vi "Get Default Instrument Configuration.vi"(0 "Instrument Handle In":refnum<k21>) -> (4 "Instrument Handle Out":refnum<k21>, 8 "Instrument Configuration":T1={"LO Sharing Mode"=enum."Automatic", "LO Routing Configurations"=[], "LO Offset Configuration"={"Mode"=enum."Automatic", "Offset (Hz)"=0.0}} {"LO Offset Configuration"."Offset (Hz)" format="%#_6p"})   [LabVIEW 2016, in "RFmxInstr.lvlib"]
uses:
  RFmxInstr.lvlib
  Instrument Configuration.ctl
  Common/Local Oscillator Sharing Mode.ctl
  Common/Local Oscillator Routing Configuration.ctl
  Common/Local Oscillator Frequency Offset Configuration.ctl
  Common/Local Oscillator Frequency Offset Mode.ctl
  <resource>/objmgr/RFmxInstr.rc
  Common/Common.lvlib
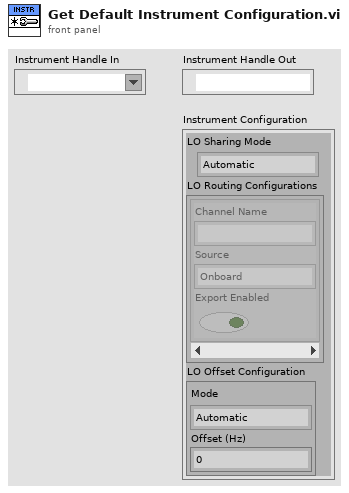
[diagram p1: front panel]
types:
  T1 = typedef "RFmxInstr.lvlib/Instrument Configuration.ctl" = cluster{"LO Sharing Mode":T2, "LO Routing Configurations":T3[], "LO Offset Configuration":T4}
  T2 = typedef "Common.lvlib/Local Oscillator Sharing Mode.ctl" = enum16{"None", "Automatic", "Manual"}
  T3 = typedef "Common.lvlib/Local Oscillator Routing Configuration.ctl" = cluster{"Channel Name":string, "Source":string, "Export Enabled":bool}
  T4 = typedef "Common.lvlib/Local Oscillator Frequency Offset Configuration.ctl" = cluster{"Mode":T5, "Offset (Hz)":dbl}
  T5 = typedef "Common.lvlib/Local Oscillator Frequency Offset Mode.ctl" = enum16{"No Offset", "Automatic", "User Defined"}
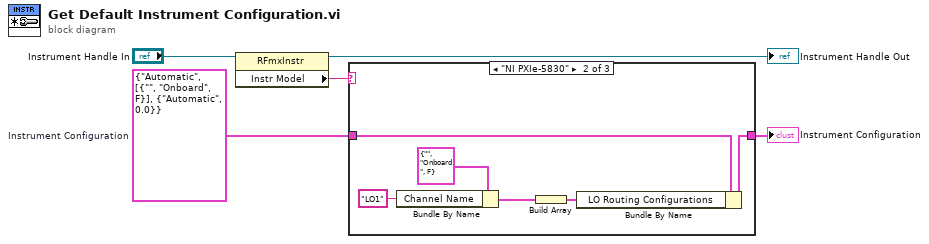
[diagram p0: block diagram]
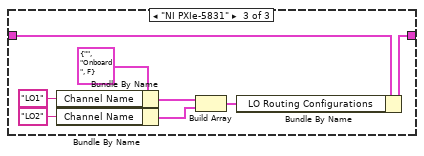
[diagram p3: hidden frame]
diagram:
  w1 = T1 {"LO Sharing Mode"=enum."Automatic", "LO Routing Configurations"=[{"Channel Name"="", "Source"="Onboard", "Export Enabled"=FALSE}], "LO Offset Configuration"={"Mode"=enum."Automatic", "Offset (Hz)"=0.0}}  # Instrument Configuration
  n1 = property class="RFmxInstr"(reference="Instrument Handle In") -> (reference out=→"Instrument Handle Out":refnum<k21>, "Instr Model"=w2:string)  [unwired: 1 in, 1 out]
  n2 = case shown="\"NI PXIe-5830\"" w2 {
    tunnel: w1 -> [w6 w11 w19]
    tunnel: [w6 w10 w18] -> w3
    frame Default {
    }
    frame "NI PXIe-5830" {
      n3 = Bundle By Name(cluster=T3 {"Channel Name"="", "Source"="Onboard", "Export Enabled"=FALSE} ("Local Oscillator Routing Configuration"), "Channel Name"="LO1") -> (w8:T3)
      n4 = Build Array(w8) -> (w7:T3[])
      n5 = Bundle By Name(cluster=w11, "LO Routing Configurations"=w7) -> (w10:T1)
    }
    frame "NI PXIe-5831" {
      w20 = T3 {"Channel Name"="", "Source"="Onboard", "Export Enabled"=FALSE} ("Local Oscillator Routing Configuration")
      n6 = Bundle By Name(cluster=w20, "Channel Name"="LO1") -> (w15:T3)
      n7 = Bundle By Name(cluster=w20, "Channel Name"="LO2") -> (w14:T3)
      n8 = Build Array(w15, w14) -> (w13:T3[])
      n9 = Bundle By Name(cluster=w19, "LO Routing Configurations"=w13) -> (w18:T1)
    }
  }
  "Instrument Configuration" <- w3
